vi "ConfigureStartupFeatures.vi"(8 "error in (no error)":errorcluster, 10 "Metric Cache":variant, 11 "Metrics":T2[](array[typedef])) -> (0 "error out":errorcluster, 2 "PFLA Feature":T1, 3 "Startup Features":T1[](array[typedef]))   [LabVIEW 2017, in "McsaStartupAnalysis.lvlib"]
uses:
  <vilib>/addons/InsightCM/Devices/Shared/Mcsa/McsaStartupAnalysis/McsaStartupAnalysis.lvlib
  <vilib>/addons/InsightCM/Devices/Shared/Mcsa/McsaStartupAnalysis/controls/StartupFeature.ctl
  <vilib>/addons/InsightCM/MessageBus/Base/controls/Metric.ctl
  <vilib>/addons/InsightCM/MessageBus/Base/controls/KeyValuePair.ctl
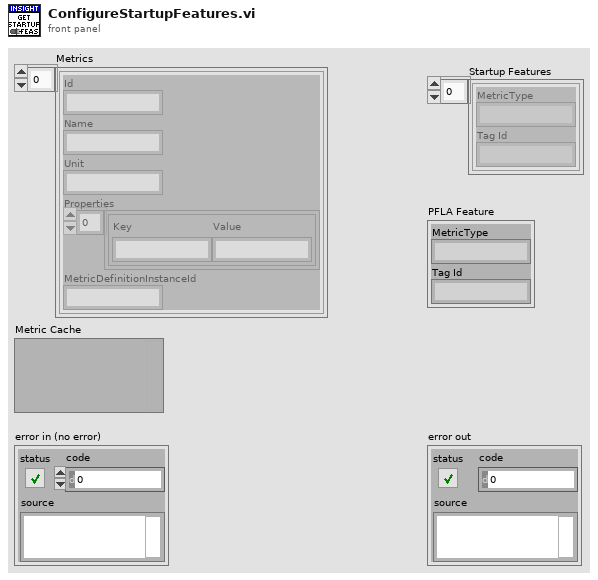
[diagram p1: front panel]
types:
  T1 = typedef "McsaStartupAnalysis.lvlib/StartupFeature.ctl" = cluster{"MetricType":string, "Tag Id":string}
  T2 = typedef "Metric.ctl" = cluster{"Id":string, "Name":string, "Unit":string, "Properties":T3[], "MetricDefinitionInstanceId":string}
  T3 = typedef "KeyValuePair.ctl" = cluster{"Key":string, "Value":string}
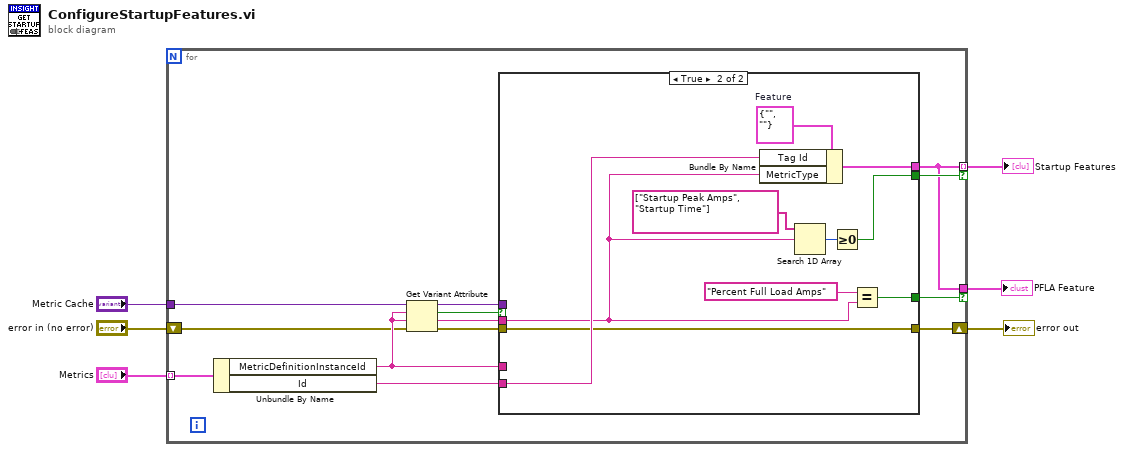
[diagram p0: block diagram]
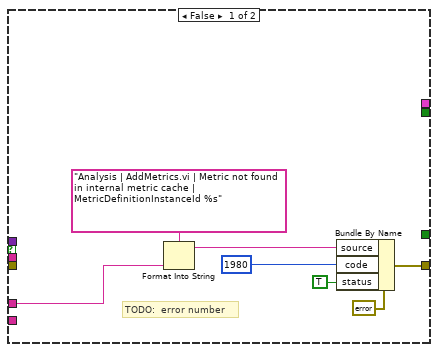
[diagram p2: hidden frame]
diagram:
  n1 = for {
    tunnel: "Metric Cache" -> [w11]
    tunnel: "Metrics" -> [w10] mode=indexing
    tunnel: [w8] -> w5 mode=indexing if=w9
    shift-right: [w15] -> w6
    shift-left: "error in (no error)" -> [w12]
    tunnel: [w8] -> w1 if=w7
    n2 = Unbundle By Name(w10) -> ("MetricDefinitionInstanceId"=w13:string, "Id"=w14:string)
    n3 = Get Variant Attribute(Variant=w11, name=w13, default value (empty Variant)=w13, error in=w12) -> (duplicate Variant=w16:variant, found=w17:bool, value=w19:string, error out=w18:errorcluster)
    n4 = case shown="True" w17 {
      tunnel: w18 -> [_ w30]
      tunnel: w19 -> [_ w28]
      tunnel: w14 -> [_ w31]
      tunnel: w16 -> [_ _]
      tunnel: [w21 w30] -> w15
      tunnel: [_ w35] -> w8
      tunnel: [_ w33] -> w9
      tunnel: w13 -> [w20 _]
      tunnel: [_ w27] -> w7
      frame False {
        # "TODO:  error number"
        n5 = Format Into String(format string="Analysis | AddMetrics.vi | Metric not found in internal metric cache | MetricDefinitionInstanceId %s" ("source"), w20) -> (resulting string=w24:string)  [unwired: 2 in, 1 out]
        n6 = Bundle By Name(cluster=errorcluster {"status"=FALSE, "code"=0, "source"=""} ("error out"), "source"=w24, "code"=1980, "status"=TRUE) -> (w21:errorcluster)
      }
      frame True {
        w36 = T1 {"MetricType"="", "Tag Id"=""}  # Feature
        n7 = Bundle By Name(cluster=w36, "Tag Id"=w31, "MetricType"=w28) -> (w35:T1)
        n8 = Search 1D Array(1D array=string[] ["Startup Peak Amps", "Startup Time"], element=w28) -> (index of element=w34:i32)  [unwired: 1 in]
        n9 = Greater Or Equal To 0?(x=w34) -> (x >= 0?=w33:bool)
        n10 = Equal?(x="Percent Full Load Amps", y=w28) -> (x = y?=w27:bool)
      }
    }
  }
  "error out" <- w6
  "Startup Features" <- w5
  "PFLA Feature" <- w1
